vi "VD-setSettings.vi"(8 "error in (no error)":errorcluster, 10 "Settings":T1, 11 "VD-LV-LiteVNA in":refnum<class "VD-LV-LiteVNA.lvclass">) -> (0 "error out":errorcluster, 3 "VD-LV-LiteVNA out":refnum<class "VD-LV-LiteVNA.lvclass">)   [LabVIEW 2020, in "VD-LV-LiteVNA.lvclass"]
uses:
  VD-LV-LiteVNA.lvclass
  VD-settings.ctl
  VD-action.ctl
  hardware-protocol/serial/HP-S-data.ctl
  VD-LV-LiteVNA.lvclass/VD-LV-LiteVNA.ctl
  hardware-protocol/serial/HP-S-Serial.lvclass
panel:
  out "Command 2":u8[][](array[numeric])
  out "Command":u8[][](array[numeric]) format="%x"
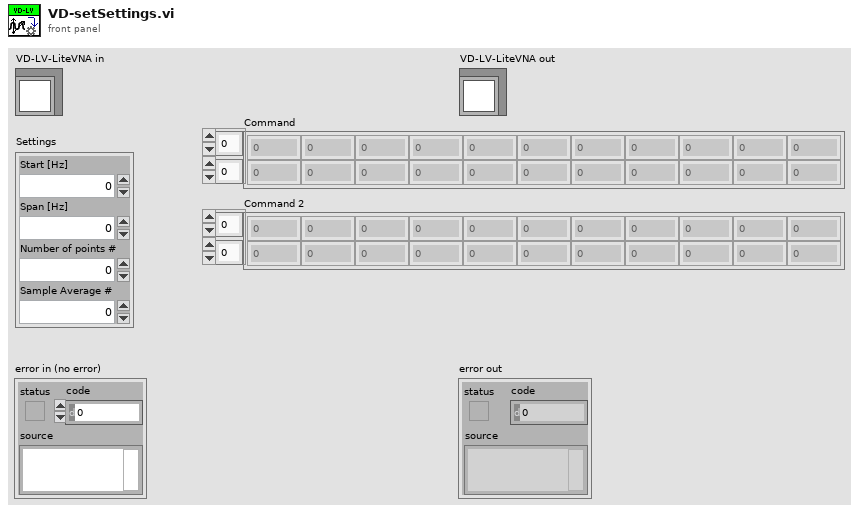
[diagram p1: front panel]
types:
  T1 = typedef "VD-LV-LiteVNA.lvclass/VD-settings.ctl" = cluster{"Start [Hz]":u64, "Span [Hz]":u64, "Number of points #":u16, "Sample Average #":u16}
  T2 = typedef "VD-LV-LiteVNA.lvclass/VD-action.ctl" = enum16{"checkCom", "SweepStartHz", "SweepStopHz", "SweepPoints", "valuesPerFrequency", "RawSamplesMode", "ValuesFIFO", "deviceVariant", "protocolVersion", "hardwareRevision", "firmwareMajor", "firmwareMinor"}
  T3 = typedef "HP-S-Serial.lvclass/HP-S-data.ctl" = u8[]
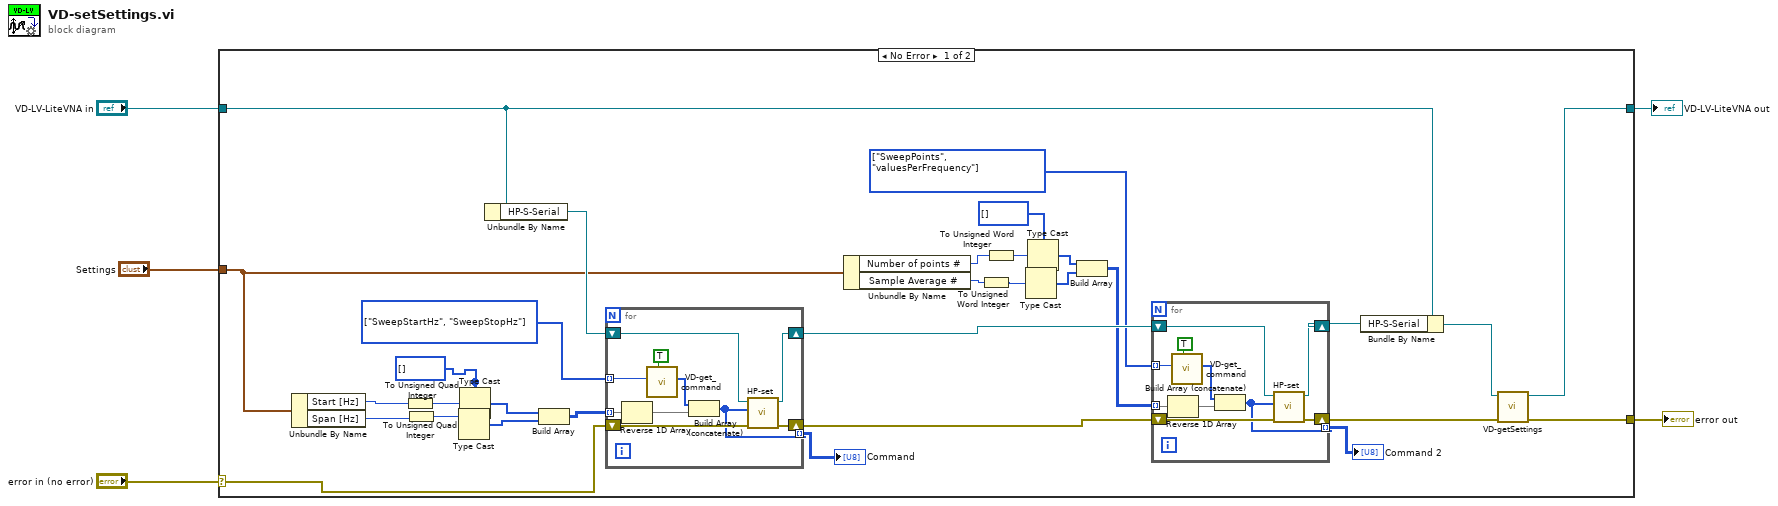
[diagram p0: block diagram]
diagram:
  n1 = case shown="No Error" "error in (no error)" {
    selector: "error in (no error)" -> [w21 w58]
    tunnel: [w8 w58] -> w4
    tunnel: [w6 w57] -> w2
    tunnel: "VD-LV-LiteVNA in" -> [w25 w57]
    tunnel: "Settings" -> [w17 _]
    frame No Error {
      w11 = T2[] [enum."SweepPoints", enum."valuesPerFrequency"] items=["checkCom", "SweepStartHz", "SweepStopHz", "SweepPoints", "valuesPerFrequency", "RawSamplesMode", "ValuesFIFO", "deviceVariant", "protocolVersion", "hardwareRevision", "firmwareMajor", "firmwareMinor"] ("Array")
      w20 = T3 [] ("8bit array")
      w24 = T3 [] ("8bit array")
      w27 = T2[] [enum."SweepStartHz", enum."SweepStopHz"] items=["checkCom", "SweepStartHz", "SweepStopHz", "SweepPoints", "valuesPerFrequency", "RawSamplesMode", "ValuesFIFO", "deviceVariant", "protocolVersion", "hardwareRevision", "firmwareMajor", "firmwareMinor"] ("Array")
      n2 = Unbundle By Name(w17) -> ("Start [Hz]"=w36:u64, "Span [Hz]"=w35:u64)
      n3 = To Unsigned Quad Integer(1:w36) -> (0:w34:u64)
      n4 = To Unsigned Quad Integer(1:w35) -> (0:w33:u64)
      n5 = Type Cast(type=w24, x=w33) -> (*(type *) &x=w29:T3)
      n6 = Type Cast(type=w24, x=w34) -> (*(type *) &x=w30:T3)
      n7 = Unbundle By Name(w25) -> ("HP-S-Serial"=w26:refnum<class "HP-S-Serial.lvclass">)
      n8 = Build Array(w30, w29) -> (w28:u8[][])
      n9 = for {
        tunnel: w28 -> [w53] mode=indexing
        tunnel: w27 -> [w56] mode=indexing
        shift-right: [w50] -> w15
        shift-left: w26 -> [w52]
        shift-right: [w51] -> w14
        shift-left: w21 -> [w49]
        tunnel: [w48] -> w16 mode=indexing
        n10 = Reverse 1D Array(array=w53) -> (reversed array=w47:u8[])
        n11 = call "VD-get_command.vi"("Write?"=TRUE, "action"=w56) -> ("Command"=w54:T3)  [unwired: 9 in]
        n12 = Build Array (concatenate)(w54, w47) -> (w48:T3)
        n13 = call-dynamic "HP-set.vi"("error in (no error)"=w49, "write buffer"=w48, "HP-S-Serial in"=w52) -> ("error out"=w51:errorcluster, "HP-S-Serial out"=w50:refnum<class "HP-S-Serial.lvclass">)  [unwired: 7 in]
      }
      "Command" <- w16
      n14 = Unbundle By Name(w17) -> ("Number of points #"=w19:u16, "Sample Average #"=w18:u16)
      n15 = To Unsigned Word Integer(number=w18) -> (unsigned 16bit integer=w31:u16)
      n16 = To Unsigned Word Integer(number=w19) -> (unsigned 16bit integer=w32:u16)
      n17 = Type Cast(type=w20, x=w31) -> (*(type *) &x=w23:T3)
      n18 = Type Cast(type=w20, x=w32) -> (*(type *) &x=w22:T3)
      n19 = Build Array(w22, w23) -> (w12:u8[][])
      n20 = for {
        tunnel: w12 -> [w43] mode=indexing
        tunnel: w11 -> [w46] mode=indexing
        shift-right: [w40] -> w13
        shift-left: w15 -> [w42]
        shift-right: [w41] -> w9
        shift-left: w14 -> [w39]
        tunnel: [w38] -> w10 mode=indexing
        n21 = Reverse 1D Array(array=w43) -> (reversed array=w37:u8[])
        n22 = call "VD-get_command.vi"("Write?"=TRUE, "action"=w46) -> ("Command"=w44:T3)  [unwired: 9 in]
        n23 = Build Array (concatenate)(w44, w37) -> (w38:T3)
        n24 = call-dynamic "HP-set.vi"("error in (no error)"=w39, "write buffer"=w38, "HP-S-Serial in"=w42) -> ("error out"=w41:errorcluster, "HP-S-Serial out"=w40:refnum<class "HP-S-Serial.lvclass">)  [unwired: 7 in]
      }
      "Command 2" <- w10
      n25 = Bundle By Name(cluster=w25, "HP-S-Serial"=w13) -> (w7:refnum<class "VD-LV-LiteVNA.lvclass">)
      n26 = call "VD-getSettings.vi"("error in (no error)"=w9, "VD-LV-LiteVNA in"=w7) -> ("error out"=w8:errorcluster, "VD-LV-LiteVNA out"=w6:refnum<class "VD-LV-LiteVNA.lvclass">)  [unwired: 7 in, 1 out]
    }
    frame Error {
    }
  }
  "error out" <- w4
  "VD-LV-LiteVNA out" <- w2
